vi "Read Accelerometer.vi"() -> ()   [LabVIEW 2011]
uses:
  LVH-EZ430.lvlib
  Private/Type Defs/EZ430-Chronos Config.ctl
panel:
  out "Accelerations":T1(graph)
  in  "Stop Button":bool
  in  "EZ430-Chronos Config":T2
  # "EZ430-Chronos Settings"
  # "Acceleration Data"
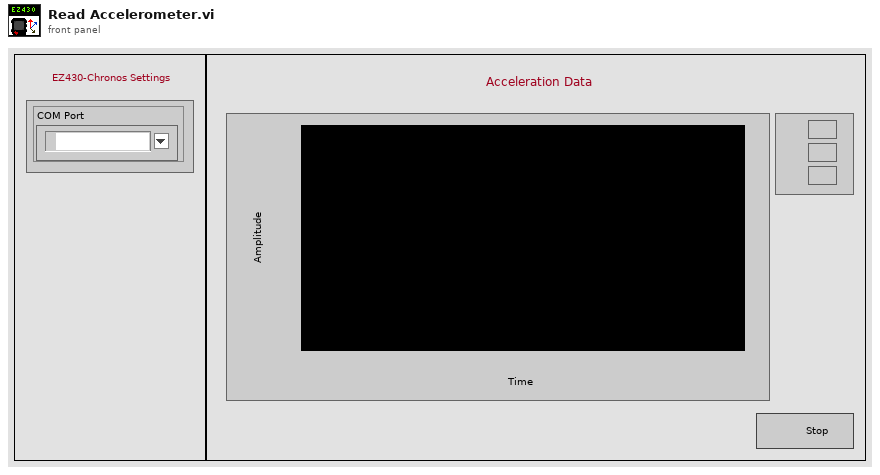
[diagram p1: front panel]
types:
  T1 = cluster{"Numeric Control":i8, "Numeric Control":i8, "Numeric Control":i8}
  T2 = typedef "LVH-EZ430.lvlib/EZ430-Chronos Config.ctl" = cluster{"COM Port":refnum<visa-resource-name>}
  T3 = typedef "LVH-EZ430.lvlib/EZ430-Chronos Ref.ctl" = cluster{"COM Port":refnum<visa-resource-name>}
  T4 = typedef "LVH-EZ430.lvlib/Accelerations.ctl" = cluster{"X Axis":i8, "Y Axis":i8, "Z Axis":i8}
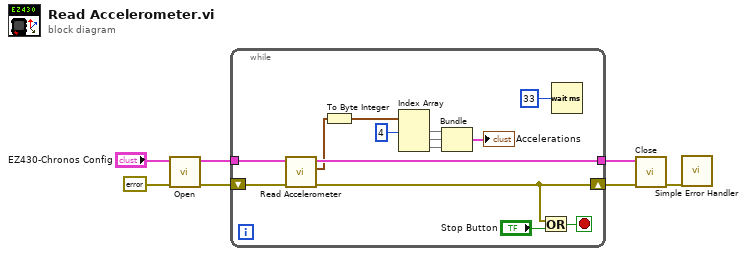
[diagram p0: block diagram]
diagram:
  n1 = call "Open.vi"("Error In"=errorcluster {"status"=FALSE, "code"=0, "source"=""}, "EZ430-Chronos Config"="EZ430-Chronos Config") -> ("Error Out"=w2:errorcluster, "EZ430-Chronos Ref"=w3:T3)  [unwired: 8 in]
  n2 = while {
    tunnel: w3 -> [w21]
    tunnel: [w19] -> w7
    shift-right: [w16] -> w4
    shift-left: w2 -> [w20]
    stop <- w18 stop-if-true
    n3 = call "Read Accelerometer.vi"("Error In"=w20, "EZ430-Chronos Ref"=w21) -> ("Error Out"=w16:errorcluster, "Accelerations"=w9:T4, "EZ430-Chronos Config"=w19:T3)  [unwired: 7 in]
    n4 = To Byte Integer(number=w9) -> (8bit integer=w10:T4)
    n5 = Index Array(array=w10, index #1=4 ("index")) -> (element #1=w13, element #2=w12, element #3=w11)  [unwired: 2 in]
    n6 = Bundle(w13, w12, w11) -> (→"Accelerations":cluster{void, void, void})  [unwired: 1 in]
    n7 = Or(x=w16, y="Stop Button") -> (x .or. y?=w18:bool)
    n8 = Wait (ms)(milliseconds to wait=u32 33) -> ()  [unwired: 1 out]
  }
  n9 = call "Close.vi"("Error In"=w4, "EZ430-Chronos Config"=w7) -> ("Error Out"=w1:errorcluster)  [unwired: 9 in]
  n10 = call <vilib>:"Simple Error Handler.vi"("error in (no error)"=w1) -> ()  [unwired: 4 in, 5 out]
